vi "NicmosGetMaskBanks.vi"(9 "error in (no error)":errorcluster caption="error out (no error)") -> (0 "READOUT out":T1=[{"MaskList"=[{"X"=6, "Y"=6, "NX"=1, "NY"=1}], "Reform X"=1, "Reform Y"=1}, {"MaskList"=[{"X"=2, "Y"=2, "NX"=9, "NY"=9}], "Reform X"=9, "Reform Y"=9}, {"MaskList"=[{"X"=48, "Y"=38, "NX"=1, "NY"=8}], "Reform X"=1, "Reform Y"=8}, {"MaskList"=[{"X"=44, "Y"=38, "NX"=8, "NY"=8}], "Reform X"=8, "Reform Y"=8}, {"MaskList"=[{"X"=14, "Y"=7, "NX"=35, "NY"=8}], "Reform X"=35, "Reform Y"=8}, {"MaskList"=[{"X"=2, "Y"=2, "NX"=100, "NY"=100}], "Reform X"=100, "Reform Y"=100}], 6 "error out":errorcluster)   [LabVIEW 2009]
uses:
  Controls/NICMOS.MASKBANKS.ctl
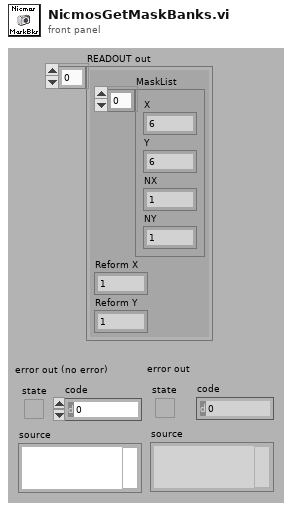
[diagram p1: front panel]
types:
  T1 = typedef "NICMOS.MASKBANKS.ctl" = cluster{"MaskList":cluster{"X":i32, "Y":i32, "NX":i32, "NY":i32}[], "Reform X":i32, "Reform Y":i32}[]
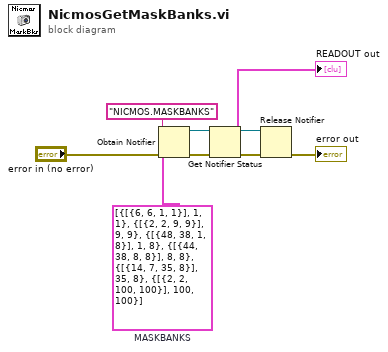
[diagram p0: block diagram]
diagram:
  w8 = T1 [{"MaskList"=[{"X"=6, "Y"=6, "NX"=1, "NY"=1}], "Reform X"=1, "Reform Y"=1}, {"MaskList"=[{"X"=2, "Y"=2, "NX"=9, "NY"=9}], "Reform X"=9, "Reform Y"=9}, {"MaskList"=[{"X"=48, "Y"=38, "NX"=1, "NY"=8}], "Reform X"=1, "Reform Y"=8}, {"MaskList"=[{"X"=44, "Y"=38, "NX"=8, "NY"=8}], "Reform X"=8, "Reform Y"=8}, {"MaskList"=[{"X"=14, "Y"=7, "NX"=35, "NY"=8}], "Reform X"=35, "Reform Y"=8}, {"MaskList"=[{"X"=2, "Y"=2, "NX"=100, "NY"=100}], "Reform X"=100, "Reform Y"=100}]  # MASKBANKS
  n1 = Obtain Notifier(name (unnamed)="NICMOS.MASKBANKS" ("nom (aucun)"), notification data type=w8, error in (no error)="error in (no error)") -> (notifier out=w1:refnum<notifier>, error out=w2:errorcluster)  [unwired: 1 in, 1 out]
  n2 = Get Notifier Status(notifier=w1, error in (no error)=w2) -> (notifier out=w4:refnum<notifier>, current notification=→"READOUT out":T1, error out=w6:errorcluster)  [unwired: 2 out]
  n3 = Release Notifier(notifier=w4, error in (no error)=w6) -> (error out=→"error out":errorcluster)  [unwired: 1 in, 2 out]
